vi "Set Gear Ratios.vi"(8 "error in (no error)":errorcluster, 11 "MF3 in":refnum<class "MF3.lvclass">) -> (0 "error out":errorcluster, 3 "MF3 out":refnum<class "MF3.lvclass">)   [LabVIEW 2011, in "MF3.lvclass"]
uses:
  MF3.lvclass
  Controls/Motor Names.ctl
  MF3.lvclass/MF3.ctl
  Finger/Finger.lvclass
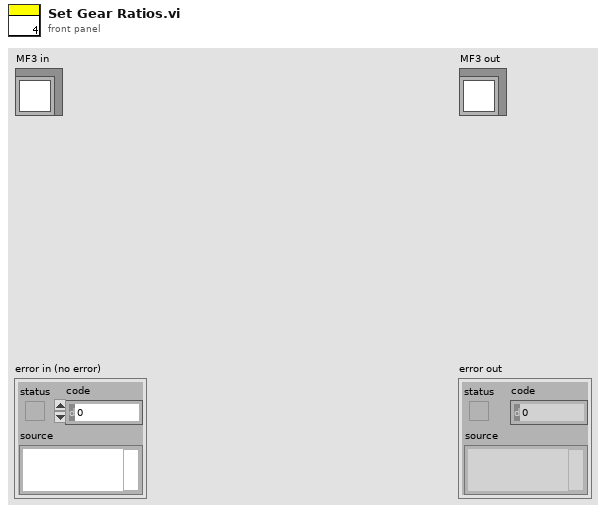
[diagram p1: front panel]
types:
  T1 = typedef "Motor Names.ctl" = enum16{"Thumb1", "Thumb2", "Thumb3", "Middle1", "Middle2", "Middle3", "Redundant", "Index1", "Index2", "Index3"}
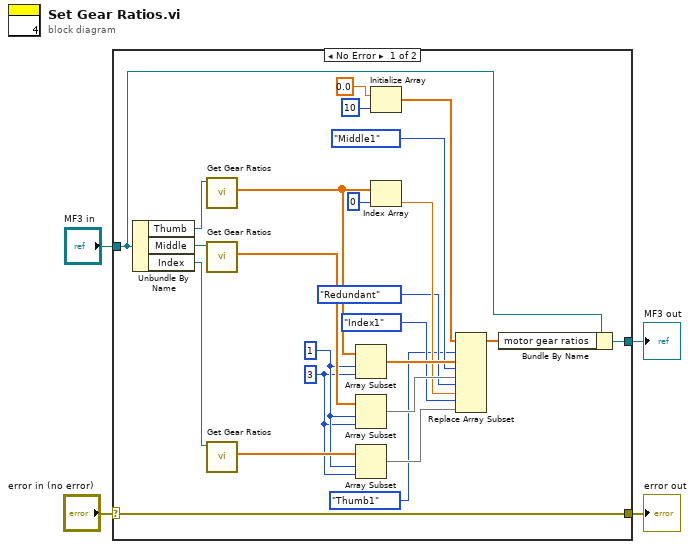
[diagram p0: block diagram]
diagram:
  n1 = case shown="No Error" "error in (no error)" {
    selector: "error in (no error)" -> [w28 w30]
    tunnel: [w28 w30] -> w3
    tunnel: [w6 w29] -> w1
    tunnel: "MF3 in" -> [w7 w29]
    frame No Error {
      w22 = 3 ("length")
      w23 = 1 ("index")
      n2 = Unbundle By Name(w7) -> ("Thumb"=w10:refnum<class "Finger.lvclass">, "Middle"=w9:refnum<class "Finger.lvclass">, "Index"=w8:refnum<class "Finger.lvclass">)
      n3 = call "Get Gear Ratios.vi"("Finger in"=w10) -> ("gear ratios"=w25:dbl[])  [unwired: 8 in, 2 out]
      n4 = call "Get Gear Ratios.vi"("Finger in"=w9) -> ("gear ratios"=w26:dbl[])  [unwired: 8 in, 2 out]
      n5 = call "Get Gear Ratios.vi"("Finger in"=w8) -> ("gear ratios"=w27:dbl[])  [unwired: 8 in, 2 out]
      n6 = Array Subset(array=w25, index=w23, length=w22) -> (w19:dbl[])
      n7 = Array Subset(array=w26, index=w23, length=w22) -> (w18:dbl[])
      n8 = Array Subset(array=w27, index=w23, length=w22) -> (w16:dbl[])
      n9 = Initialize Array(0.0 ("element"), 10 ("dimension size")) -> (w11:dbl[])
      n10 = Index Array(array=w25, index=0) -> (element=w17:dbl)
      n11 = Replace Array Subset(array=w11, new element #1=w19, index #1=Motor_Names."Thumb1" ("Motor Names"), new element #2=w18, index #2=Motor_Names."Middle1" ("Motor Names"), new element #3=w17, index #3=Motor_Names."Redundant" ("Motor Names"), new element #4=w16, index #4=Motor_Names."Index1" ("Motor Names")) -> (w5:dbl[])
      n12 = Bundle By Name(cluster=w7, "motor gear ratios"=w5) -> (w6:refnum<class "MF3.lvclass">)
    }
    frame Error {
    }
  }
  "error out" <- w3
  "MF3 out" <- w1
